vi "Mensaje arrive.vi"(8 "error in (no error)":errorcluster, 10 "Palabra entrada":string, 11 "Mensajes in":refnum<class "Mensajes.lvclass">) -> (0 "error out":errorcluster, 3 "Mensajes out":refnum<class "Mensajes.lvclass">)   [LabVIEW 2021, in "Mensajes.lvlib" / "Mensajes.lvclass"]
uses:
  Mensajes.lvclass
  Mensajes.lvclass/Mensajes.ctl
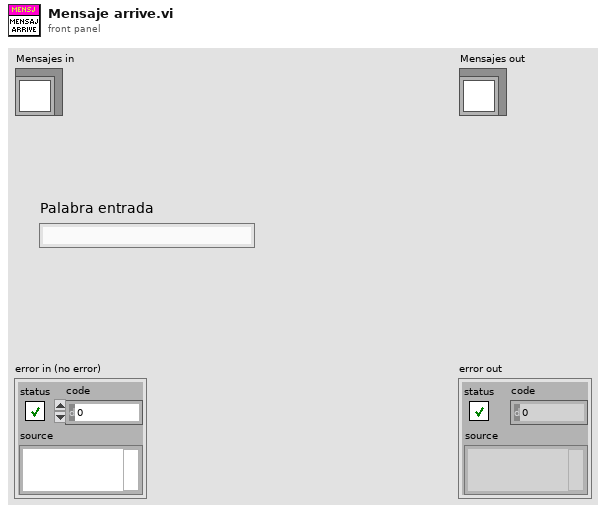
[diagram p1: front panel]
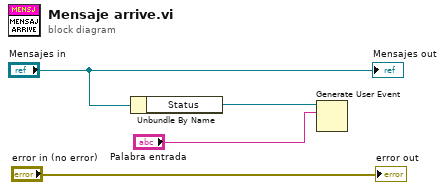
[diagram p0: block diagram]
diagram:
  n1 = Unbundle By Name("Mensajes in") -> ("Status"=w2:refnum<user-event>)
  n2 = Generate User Event(user event=w2, event data cluster="Palabra entrada") -> ()  [unwired: 2 in, 2 out]
  "error out" <- "error in (no error)"
  "Mensajes out" <- "Mensajes in"
